vi "Game.vi"() -> ()   [LabVIEW 2018]
uses:
  Control 1.ctl
  Control 2.ctl
panel:
  in  "Switch Player":bool
  in  "End Game":bool
  in  "Cluster":T1
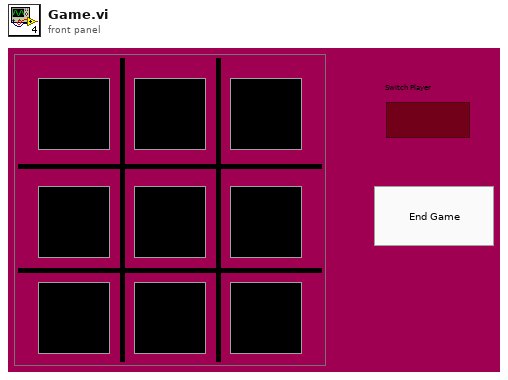
[diagram p1: front panel]
types:
  T1 = typedef "Control 1.ctl" = cluster{"OK Button":bool, "OK Button 2":bool, "OK Button 3":bool, "OK Button 4":bool, "OK Button 5":bool, "OK Button 6":bool, "OK Button 7":bool, "OK Button 8":bool, "OK Button 9":bool}
  T2 = typedef "Control 2.ctl" = enum16{"Init", "Move", "Check O", "Check X", "Winner O", "Winner X", "End"}
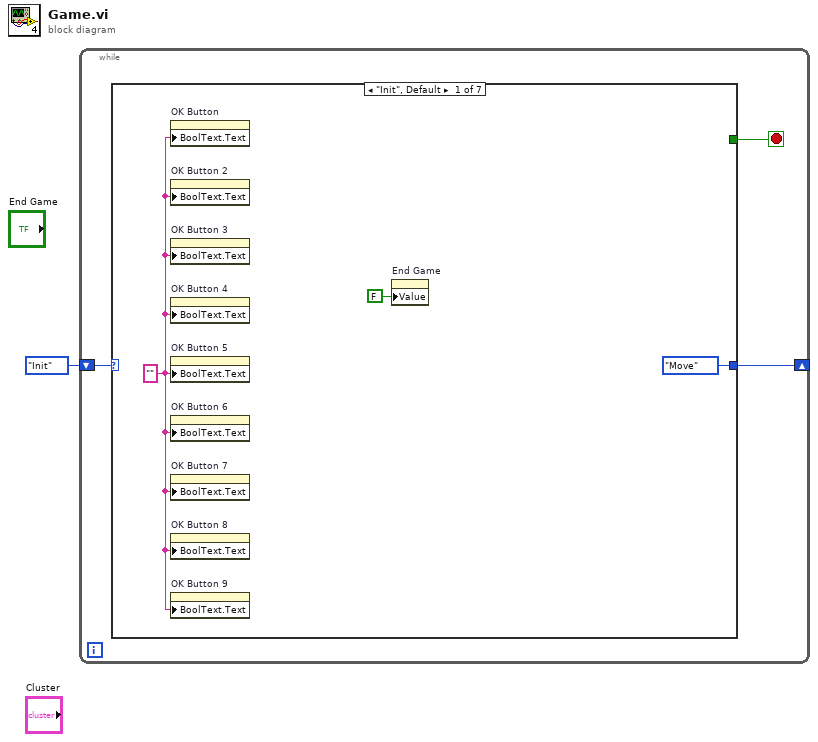
[diagram p0: block diagram]
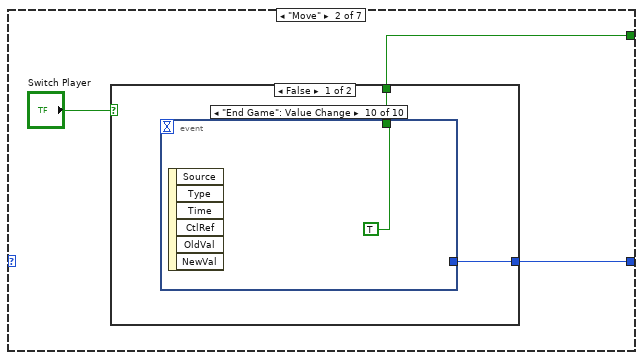
[diagram p2: hidden frame]
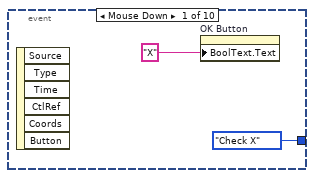
[diagram p3: hidden frame]
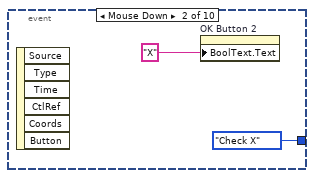
[diagram p4: hidden frame]
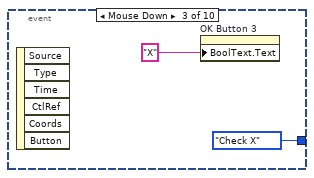
[diagram p5: hidden frame]
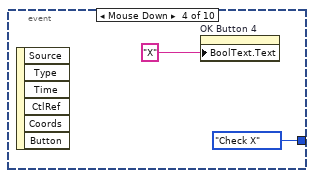
[diagram p6: hidden frame]
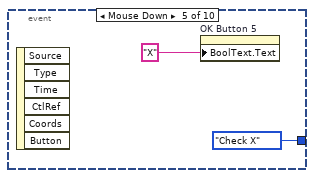
[diagram p7: hidden frame]
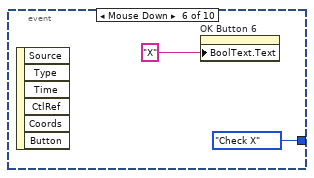
[diagram p8: hidden frame]
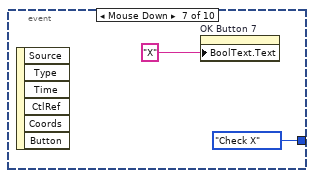
[diagram p9: hidden frame]
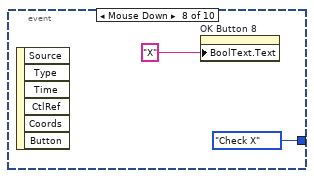
[diagram p10: hidden frame]
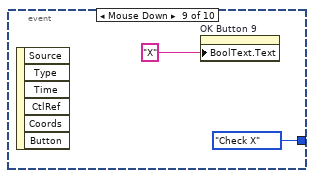
[diagram p11: hidden frame]
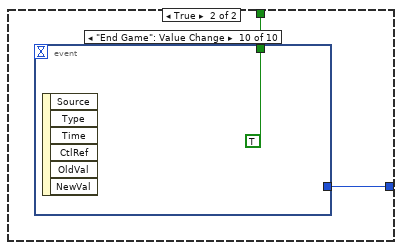
[diagram p12: hidden frame]
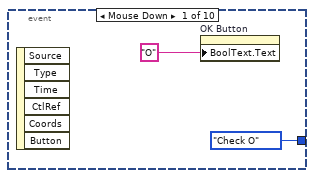
[diagram p13: hidden frame]
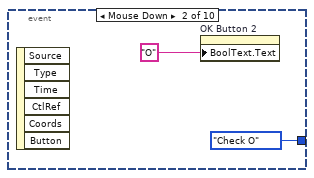
[diagram p14: hidden frame]
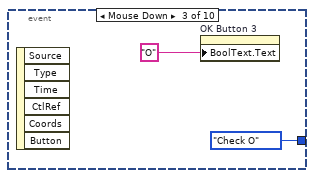
[diagram p15: hidden frame]
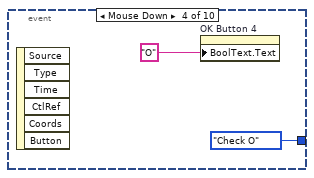
[diagram p16: hidden frame]
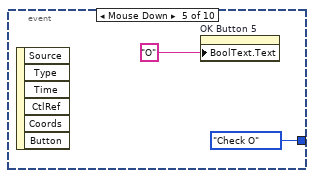
[diagram p17: hidden frame]
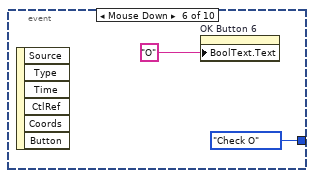
[diagram p18: hidden frame]
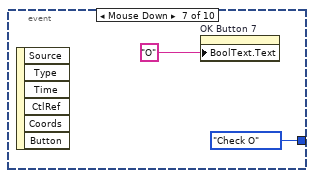
[diagram p19: hidden frame]
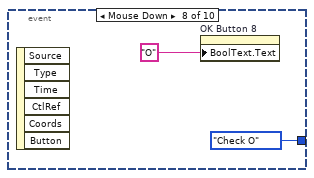
[diagram p20: hidden frame]
diagram:
  n1 = while {
    shift-right: [w3] -> _
    shift-left: Control_2."Init" -> [w4]
    stop <- w2 stop-if-true
    n2 = case shown="\"Init\", Default" w4 {
      tunnel: [Control_2."Move" w9 w72 w93 Control_2."End" Control_2."End" Control_2."Init"] -> w3
      tunnel: [_ w8 _ _ _ _ _] -> w2
      frame "Init", Default {
        w7 = ""
        n3 = property on="OK Button" class="Bool (strict)"("BoolText.Text"=w7) -> ()  [unwired: 2 in, 2 out]
        n4 = property on="OK Button 2" class="Bool (strict)"("BoolText.Text"=w7) -> ()  [unwired: 2 in, 2 out]
        n5 = property on="OK Button 3" class="Bool (strict)"("BoolText.Text"=w7) -> ()  [unwired: 2 in, 2 out]
        n6 = property on="OK Button 4" class="Bool (strict)"("BoolText.Text"=w7) -> ()  [unwired: 2 in, 2 out]
        n7 = property on="OK Button 5" class="Bool (strict)"("BoolText.Text"=w7) -> ()  [unwired: 2 in, 2 out]
        n8 = property on="OK Button 6" class="Bool (strict)"("BoolText.Text"=w7) -> ()  [unwired: 2 in, 2 out]
        n9 = property on="OK Button 7" class="Bool (strict)"("BoolText.Text"=w7) -> ()  [unwired: 2 in, 2 out]
        n10 = property on="OK Button 8" class="Bool (strict)"("BoolText.Text"=w7) -> ()  [unwired: 2 in, 2 out]
        n11 = property on="OK Button 9" class="Bool (strict)"("BoolText.Text"=w7) -> ()  [unwired: 2 in, 2 out]
        n12 = property on="End Game" class="Bool (strict)"("Value"=FALSE ("End Game")) -> ()  [unwired: 2 in, 2 out]
      }
      frame "Move" {
        n13 = case shown="False" "Switch Player" {
          tunnel: [w12 w33] -> w9
          tunnel: [w11 w32] -> w8
          frame False {
            n14 = event shown="[9] \"End Game\": Value Change" {
              selector: _ -> [_ _ _ _ _ _ _ _ _ _]
              dyn-events: _ -> [_ _ _ _ _ _ _ _ _ _]
              timeout: _ -> [_ _ _ _ _ _ _ _ _ _]
              tunnel: [Control_2."Check X" Control_2."Check X" Control_2."Check X" Control_2."Check X" Control_2."Check X" Control_2."Check X" Control_2."Check X" Control_2."Check X" Control_2."Check X" _] -> w12
              tunnel: [_ _ _ _ _ _ _ _ _ TRUE] -> w11
              event Mouse Down {
                n15 = event-data() -> ()  [unwired: 1 in, 6 out]
                n16 = property on="OK Button" class="Bool (strict)"("BoolText.Text"="X" ("Boolean Text.Text")) -> ()  [unwired: 2 in, 2 out]
              }
              event Mouse Down {
                n17 = event-data() -> ()  [unwired: 1 in, 6 out]
                n18 = property on="OK Button 2" class="Bool (strict)"("BoolText.Text"="X" ("Boolean Text.Text")) -> ()  [unwired: 2 in, 2 out]
              }
              event Mouse Down {
                n19 = event-data() -> ()  [unwired: 1 in, 6 out]
                n20 = property on="OK Button 3" class="Bool (strict)"("BoolText.Text"="X" ("Boolean Text.Text")) -> ()  [unwired: 2 in, 2 out]
              }
              event Mouse Down {
                n21 = event-data() -> ()  [unwired: 1 in, 6 out]
                n22 = property on="OK Button 4" class="Bool (strict)"("BoolText.Text"="X" ("Boolean Text.Text")) -> ()  [unwired: 2 in, 2 out]
              }
              event Mouse Down {
                n23 = event-data() -> ()  [unwired: 1 in, 6 out]
                n24 = property on="OK Button 5" class="Bool (strict)"("BoolText.Text"="X" ("Boolean Text.Text")) -> ()  [unwired: 2 in, 2 out]
              }
              event Mouse Down {
                n25 = event-data() -> ()  [unwired: 1 in, 6 out]
                n26 = property on="OK Button 6" class="Bool (strict)"("BoolText.Text"="X" ("Boolean Text.Text")) -> ()  [unwired: 2 in, 2 out]
              }
              event Mouse Down {
                n27 = event-data() -> ()  [unwired: 1 in, 6 out]
                n28 = property on="OK Button 7" class="Bool (strict)"("BoolText.Text"="X" ("Boolean Text.Text")) -> ()  [unwired: 2 in, 2 out]
              }
              event Mouse Down {
                n29 = event-data() -> ()  [unwired: 1 in, 6 out]
                n30 = property on="OK Button 8" class="Bool (strict)"("BoolText.Text"="X" ("Boolean Text.Text")) -> ()  [unwired: 2 in, 2 out]
              }
              event Mouse Down {
                n31 = event-data() -> ()  [unwired: 1 in, 6 out]
                n32 = property on="OK Button 9" class="Bool (strict)"("BoolText.Text"="X" ("Boolean Text.Text")) -> ()  [unwired: 2 in, 2 out]
              }
              event "End Game": Value Change {
                n33 = event-data() -> ()  [unwired: 1 in, 6 out]
              }
            }
          }
          frame True {
            n34 = event shown="[9] \"End Game\": Value Change" {
              selector: _ -> [_ _ _ _ _ _ _ _ _ _]
              dyn-events: _ -> [_ _ _ _ _ _ _ _ _ _]
              timeout: _ -> [_ _ _ _ _ _ _ _ _ _]
              tunnel: [Control_2."Check O" Control_2."Check O" Control_2."Check O" Control_2."Check O" Control_2."Check O" Control_2."Check O" Control_2."Check O" Control_2."Check O" Control_2."Check O" _] -> w33
              tunnel: [_ _ _ _ _ _ _ _ _ TRUE] -> w32
              event Mouse Down {
                n35 = event-data() -> ()  [unwired: 1 in, 6 out]
                n36 = property on="OK Button" class="Bool (strict)"("BoolText.Text"="O") -> ()  [unwired: 2 in, 2 out]
              }
              event Mouse Down {
                n37 = event-data() -> ()  [unwired: 1 in, 6 out]
                n38 = property on="OK Button 2" class="Bool (strict)"("BoolText.Text"="O" ("Boolean Text.Text")) -> ()  [unwired: 2 in, 2 out]
              }
              event Mouse Down {
                n39 = event-data() -> ()  [unwired: 1 in, 6 out]
                n40 = property on="OK Button 3" class="Bool (strict)"("BoolText.Text"="O" ("Boolean Text.Text")) -> ()  [unwired: 2 in, 2 out]
              }
              event Mouse Down {
                n41 = event-data() -> ()  [unwired: 1 in, 6 out]
                n42 = property on="OK Button 4" class="Bool (strict)"("BoolText.Text"="O" ("Boolean Text.Text")) -> ()  [unwired: 2 in, 2 out]
              }
              event Mouse Down {
                n43 = event-data() -> ()  [unwired: 1 in, 6 out]
                n44 = property on="OK Button 5" class="Bool (strict)"("BoolText.Text"="O" ("Boolean Text.Text")) -> ()  [unwired: 2 in, 2 out]
              }
              event Mouse Down {
                n45 = event-data() -> ()  [unwired: 1 in, 6 out]
                n46 = property on="OK Button 6" class="Bool (strict)"("BoolText.Text"="O" ("Boolean Text.Text")) -> ()  [unwired: 2 in, 2 out]
              }
              event Mouse Down {
                n47 = event-data() -> ()  [unwired: 1 in, 6 out]
                n48 = property on="OK Button 7" class="Bool (strict)"("BoolText.Text"="O" ("Boolean Text.Text")) -> ()  [unwired: 2 in, 2 out]
              }
              event Mouse Down {
                n49 = event-data() -> ()  [unwired: 1 in, 6 out]
                n50 = property on="OK Button 8" class="Bool (strict)"("BoolText.Text"="O" ("Boolean Text.Text")) -> ()  [unwired: 2 in, 2 out]
              }
              event Mouse Down {
                n51 = event-data() -> ()  [unwired: 1 in, 6 out]
                n52 = property on="OK Button 9" class="Bool (strict)"("BoolText.Text"="O" ("Boolean Text.Text")) -> ()  [unwired: 2 in, 2 out]
              }
              event "End Game": Value Change {
                n53 = event-data() -> ()  [unwired: 1 in, 6 out]
              }
            }
          }
        }
      }
      frame "Check O" {
        n54 = property on="OK Button 2" class="Bool (strict)"() -> ("BoolText.Text"=w66:string)  [unwired: 2 in, 2 out]
        n55 = property on="OK Button 4" class="Bool (strict)"() -> ("BoolText.Text"=w68:string)  [unwired: 2 in, 2 out]
        n56 = property on="OK Button" class="Bool (strict)"() -> ("BoolText.Text"=w61:string)  [unwired: 2 in, 2 out]
        n57 = property on="OK Button 6" class="Bool (strict)"() -> ("BoolText.Text"=w63:string)  [unwired: 2 in, 2 out]
        n58 = property on="OK Button 8" class="Bool (strict)"() -> ("BoolText.Text"=w65:string)  [unwired: 2 in, 2 out]
        n59 = property on="OK Button 7" class="Bool (strict)"() -> ("BoolText.Text"=w56:string)  [unwired: 2 in, 2 out]
        n60 = property on="OK Button 3" class="Bool (strict)"() -> ("BoolText.Text"=w58:string)  [unwired: 2 in, 2 out]
        n61 = property on="OK Button 5" class="Bool (strict)"() -> ("BoolText.Text"=w57:string)  [unwired: 2 in, 2 out]
        n62 = property on="OK Button 9" class="Bool (strict)"() -> ("BoolText.Text"=w60:string)  [unwired: 2 in, 2 out]
        n63 = call "CheckO.vi"("BoolText.Text"=w58, "BoolText.Text 2"=w66, "BoolText.Text 3"=w61) -> ("Boolean"=w71:bool)  [unwired: 8 in]
        n64 = call "CheckO.vi"("BoolText.Text"=w56, "BoolText.Text 2"=w68, "BoolText.Text 3"=w61) -> ("Boolean"=w67:bool)  [unwired: 8 in]
        n65 = call "CheckO.vi"("BoolText.Text"=w60, "BoolText.Text 2"=w63, "BoolText.Text 3"=w58) -> ("Boolean"=w62:bool)  [unwired: 8 in]
        n66 = call "CheckO.vi"("BoolText.Text"=w60, "BoolText.Text 2"=w65, "BoolText.Text 3"=w56) -> ("Boolean"=w69:bool)  [unwired: 8 in]
        n67 = call "CheckO.vi"("BoolText.Text"=w63, "BoolText.Text 2"=w57, "BoolText.Text 3"=w68) -> ("Boolean"=w70:bool)  [unwired: 8 in]
        n68 = call "CheckO.vi"("BoolText.Text"=w65, "BoolText.Text 2"=w57, "BoolText.Text 3"=w66) -> ("Boolean"=w64:bool)  [unwired: 8 in]
        n69 = call "CheckO.vi"("BoolText.Text"=w60, "BoolText.Text 2"=w57, "BoolText.Text 3"=w61) -> ("Boolean"=w59:bool)  [unwired: 8 in]
        n70 = call "CheckO.vi"("BoolText.Text"=w56, "BoolText.Text 2"=w57, "BoolText.Text 3"=w58) -> ("Boolean"=w53:bool)  [unwired: 8 in]
        n71 = Build Array(w71, w70, w69, w67, w64, w62, w59, w53) -> (w55:bool[])
        n72 = Or Array Elements(Boolean array=w55) -> (logical OR=w54:bool)
        n73 = Select(t=Control_2."Winner O", s=w54, f=Control_2."Move") -> (s? t:f=w72:T2)
      }
      frame "Check X" {
        n74 = property on="OK Button 2" class="Bool (strict)"() -> ("BoolText.Text"=w91:string)  [unwired: 2 in, 2 out]
        n75 = property on="OK Button 4" class="Bool (strict)"() -> ("BoolText.Text"=w92:string)  [unwired: 2 in, 2 out]
        n76 = property on="OK Button" class="Bool (strict)"() -> ("BoolText.Text"=w88:string)  [unwired: 2 in, 2 out]
        n77 = property on="OK Button 7" class="Bool (strict)"() -> ("BoolText.Text"=w84:string)  [unwired: 2 in, 2 out]
        n78 = property on="OK Button 6" class="Bool (strict)"() -> ("BoolText.Text"=w89:string)  [unwired: 2 in, 2 out]
        n79 = property on="OK Button 8" class="Bool (strict)"() -> ("BoolText.Text"=w90:string)  [unwired: 2 in, 2 out]
        n80 = property on="OK Button 5" class="Bool (strict)"() -> ("BoolText.Text"=w85:string)  [unwired: 2 in, 2 out]
        n81 = property on="OK Button 3" class="Bool (strict)"() -> ("BoolText.Text"=w86:string)  [unwired: 2 in, 2 out]
        n82 = property on="OK Button 9" class="Bool (strict)"() -> ("BoolText.Text"=w87:string)  [unwired: 2 in, 2 out]
        n83 = call "CheckX.vi"("BoolText.Text"=w86, "BoolText.Text 2"=w91, "BoolText.Text 3"=w88) -> ("Boolean"=w83:bool)  [unwired: 8 in]
        n84 = call "CheckX.vi"("BoolText.Text"=w84, "BoolText.Text 2"=w92, "BoolText.Text 3"=w88) -> ("Boolean"=w81:bool)  [unwired: 8 in]
        n85 = call "CheckX.vi"("BoolText.Text"=w87, "BoolText.Text 2"=w89, "BoolText.Text 3"=w86) -> ("Boolean"=w78:bool)  [unwired: 8 in]
        n86 = call "CheckX.vi"("BoolText.Text"=w87, "BoolText.Text 2"=w90, "BoolText.Text 3"=w84) -> ("Boolean"=w79:bool)  [unwired: 8 in]
        n87 = call "CheckX.vi"("BoolText.Text"=w89, "BoolText.Text 2"=w85, "BoolText.Text 3"=w92) -> ("Boolean"=w82:bool)  [unwired: 8 in]
        n88 = call "CheckX.vi"("BoolText.Text"=w90, "BoolText.Text 2"=w85, "BoolText.Text 3"=w91) -> ("Boolean"=w80:bool)  [unwired: 8 in]
        n89 = call "CheckX.vi"("BoolText.Text"=w87, "BoolText.Text 2"=w85, "BoolText.Text 3"=w88) -> ("Boolean"=w77:bool)  [unwired: 8 in]
        n90 = call "CheckX.vi"("BoolText.Text"=w84, "BoolText.Text 2"=w85, "BoolText.Text 3"=w86) -> ("Boolean"=w76:bool)  [unwired: 8 in]
        n91 = Build Array(w83, w82, w81, w80, w79, w78, w77, w76) -> (w75:bool[])
        n92 = Or Array Elements(Boolean array=w75) -> (logical OR=w96:bool)
        n93 = Select(t=Control_2."Winner X", s=w96, f=Control_2."Move") -> (s? t:f=w93:T2)
      }
      frame "Winner O" {
        n94 = One Button Dialog(message="Winner: Player O") -> ()  [unwired: 1 in, 1 out]
      }
      frame "Winner X" {
        n95 = One Button Dialog(message="Winner: Player X") -> ()  [unwired: 1 in, 1 out]
      }
      frame "End" {
      }
    }
  }
